vi "compileScript.vi"(8 "error in (no error)":errorcluster, 9 "current time":timestamp, 10 "Path":path, 11 "CompiledList in":refnum<class "CompiledList.lvclass">) -> (0 "error out":errorcluster, 3 "CompiledList out":refnum<class "CompiledList.lvclass">)   [LabVIEW 2011, in "Compiler.lvlib" / "CompiledList.lvclass"]
uses:
  CompiledList.lvclass
  Hal/Channels/DDSOutput/Generic/DDSOutput.lvclass
  Hal/Channels/Digital/DigitalOutput.lvclass
  Hal/Channels/VoltOutput/AnalogOutput.lvclass
  DataMappers/DeviceData/DeviceData.lvclass
  DataMappers/DeviceData/DoDeviceData/DoDeviceData.lvclass
  DataMappers/DeviceData/AoDeviceData/AoDeviceData.lvclass
  DataMappers/DeviceData/RfOutputData/RfOutputData.lvclass
  ScriptListCompiler/ScriptListCompiler.lvclass
  DatabaseHelpers/Database Objects/DeviceArray/DeviceArray.lvclass
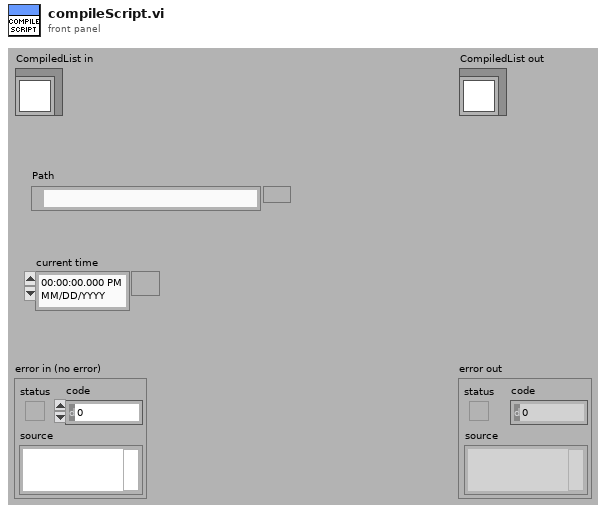
[diagram p1: front panel]
types:
  T1 = enum16{"digitalOutput", "digitalInput", "analogOutput", "analogInput", "rfOutput", "ethernetSupply"}
  T2 = cluster{"ScriptListCompiler out":refnum<class "ScriptListCompiler.lvclass">, refnum<class "AnalogOutput.lvclass">[], refnum<class "DigitalOutput.lvclass">[], refnum<class "DDSOutput.lvclass">[]}
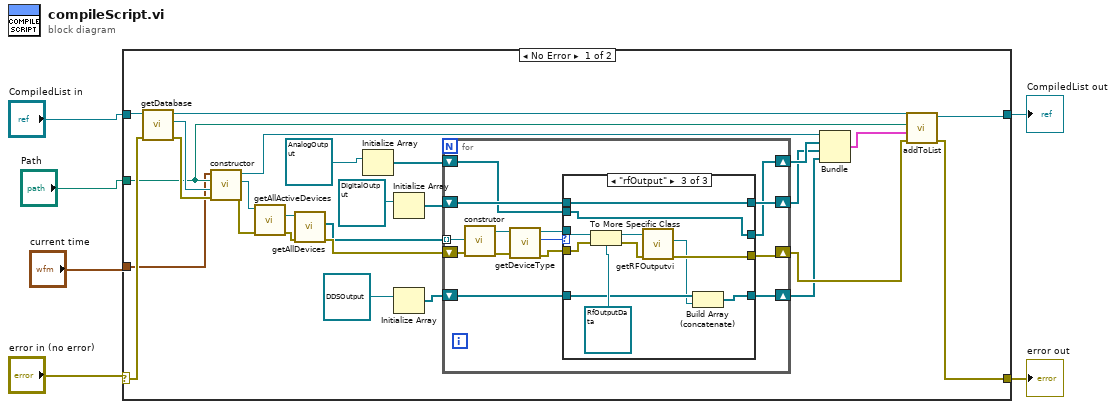
[diagram p0: block diagram]
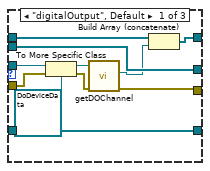
[diagram p2: hidden frame]
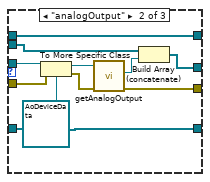
[diagram p3: hidden frame]
diagram:
  n1 = case shown="No Error" "error in (no error)" {
    selector: "error in (no error)" -> [w20 w82]
    tunnel: [w11 w82] -> w2
    tunnel: [w15 w81] -> w3
    tunnel: "CompiledList in" -> [w23 w81]
    tunnel: "Path" -> [w13 _]
    tunnel: "current time" -> [w10 _]
    frame No Error {
      n2 = call "getDatabase.vi"("error in (no error)"=w20, "CompiledList in"=w23) -> ("error out"=w21:errorcluster, "deviceDataBase out"=w22:refnum<class "deviceDataBase.lvclass">, "CompiledList out"=w16:refnum<class "CompiledList.lvclass">)  [unwired: 7 in]
      n3 = call "constructor.vi"("error in (no error)"=w21, "deviceDataBase"=w22, "Path"=w13, "compiledTime"=w10) -> ("error out"=w30:errorcluster, "DeviceArray"=w33:refnum<class "DeviceArray.lvclass">, "ScriptListCompiler out"=w19:refnum<class "ScriptListCompiler.lvclass">)  [unwired: 4 in, 1 out]
      n4 = call "getAllActiveDevices.vi"("error in (no error)"=w30, "DeviceArray in"=w33) -> ("error out"=w31:errorcluster, "DeviceArray"=w32:refnum<class "DeviceArray.lvclass">)  [unwired: 7 in, 1 out]
      n5 = call "getAllDevices.vi"("error in (no error)"=w31, "DeviceArray.lvclass in"=w32) -> ("error out"=w29:errorcluster, "deviceArray"=w28:refnum<class "device.lvclass">[])  [unwired: 7 in, 1 out]
      n6 = Initialize Array(refnum<class "AnalogOutput.lvclass"> refnum ("aOChannel")) -> (w26:refnum<class "AnalogOutput.lvclass">[])  [unwired: 1 in]
      n7 = Initialize Array(refnum<class "DigitalOutput.lvclass"> refnum ("DigitalOutput")) -> (w25:refnum<class "DigitalOutput.lvclass">[])  [unwired: 1 in]
      n8 = Initialize Array(refnum<class "DDSOutput.lvclass"> refnum ("Hardware:Channels.lvlib:DDSOutput.lvclass")) -> (w8:refnum<class "DDSOutput.lvclass">[])  [unwired: 1 in]
      n9 = for {
        shift-right: [w37] -> w12
        shift-left: w29 -> [w47]
        shift-right: [w42] -> w17
        shift-left: w25 -> [w41]
        shift-right: [w40] -> w18
        shift-left: w26 -> [w39]
        tunnel: w28 -> [w36] mode=indexing
        shift-right: [w34] -> w7
        shift-left: w8 -> [w35]
        n10 = call "construtor.vi"("error in (no error)"=w47, "device"=w36) -> ("error out"=w46:errorcluster, "DeviceData out"=w45:refnum<class "DeviceData.lvclass">)  [unwired: 8 in]
        n11 = call-dynamic "getDeviceType.vi"("error in (no error)"=w46, "DeviceData in"=w45) -> ("error out"=w38:errorcluster, "type"=w44:T1, "DeviceData out"=w43:refnum<class "DeviceData.lvclass">)  [unwired: 7 in]
        n12 = case shown="\"rfOutput\"" w44 {
          tunnel: w43 -> [w58 w68 w77]
          tunnel: [w51 w65 w80] -> w42
          tunnel: w41 -> [w50 w65 w80]
          tunnel: [w55 w60 w74] -> w40
          tunnel: w39 -> [w55 w62 w74]
          tunnel: w38 -> [w54 w64 w75]
          tunnel: [w52 w63 w73] -> w37
          tunnel: w35 -> [w48 w59 w72]
          tunnel: [w48 w59 w71] -> w34
          frame "digitalOutput", Default {
            n13 = To More Specific Class(target class=refnum<class "DoDeviceData.lvclass"> refnum ("DoDeviceData.lvclass in"), reference=w58, error in=w54) -> (specific class reference=w56:refnum<class "DoDeviceData.lvclass">, error out=w53:errorcluster)
            n14 = call "getDOChannel.vi"("error in (no error)"=w53, "DoDeviceData.lvclass in"=w56) -> ("error out"=w52:errorcluster, "DigitalOutput"=w49:refnum<class "DigitalOutput.lvclass">)  [unwired: 7 in, 1 out]
            n15 = Build Array (concatenate)(w50, w49) -> (w51:refnum<class "DigitalOutput.lvclass">[])
          }
          frame "analogOutput" {
            n16 = To More Specific Class(target class=refnum<class "AoDeviceData.lvclass"> refnum ("AoDeviceData.lvclass in"), reference=w68, error in=w64) -> (specific class reference=w66:refnum<class "AoDeviceData.lvclass">, error out=w69:errorcluster)
            n17 = call "getAnalogOutput.vi"("error in (no error)"=w69, "AoDeviceData.lvclass in"=w66) -> ("error out"=w63:errorcluster, "aOChannel"=w61:refnum<class "AnalogOutput.lvclass">)  [unwired: 7 in, 1 out]
            n18 = Build Array (concatenate)(w62, w61) -> (w60:refnum<class "AnalogOutput.lvclass">[])
          }
          frame "rfOutput" {
            n19 = To More Specific Class(target class=refnum<class "RfOutputData.lvclass"> refnum ("DataMappers.lvlib:RfOutputData.lvclass"), reference=w77, error in=w75) -> (specific class reference=w79:refnum<class "RfOutputData.lvclass">, error out=w78:errorcluster)
            n20 = call-dynamic "getRFOutputvi.vi"("error in (no error)"=w78, "RfOutputData in"=w79) -> ("error out"=w73:errorcluster, "DDSOutput"=w70:refnum<class "DDSOutput.lvclass">)  [unwired: 7 in, 1 out]
            n21 = Build Array (concatenate)(w72, w70) -> (w71:refnum<class "DDSOutput.lvclass">[])
          }
        }
      }
      n22 = Bundle("ScriptListCompiler out"=w19, w18, w17, w7) -> (w14:T2)  [unwired: 1 in]
      n23 = call "addToList.vi"("error in (no error)"=w12, "CompiledScript"=w14, "Path"=w13, "CompiledList in"=w16) -> ("error out"=w11:errorcluster, "CompiledList out"=w15:refnum<class "CompiledList.lvclass">)  [unwired: 6 in]
    }
    frame Error {
    }
  }
  "error out" <- w2
  "CompiledList out" <- w3
